vi "Read id.vi"(8 "error in (no error)":errorcluster, 11 "Electrometer in":refnum<class "Electrometer.lvclass">) -> (0 "error out":errorcluster, 2 "ElectrometerId":enum16{"", "ID1", "ID2"}(ring), 3 "Electrometer out":refnum<class "Electrometer.lvclass">)   [LabVIEW 2016]
uses:
  Electrometer.lvclass
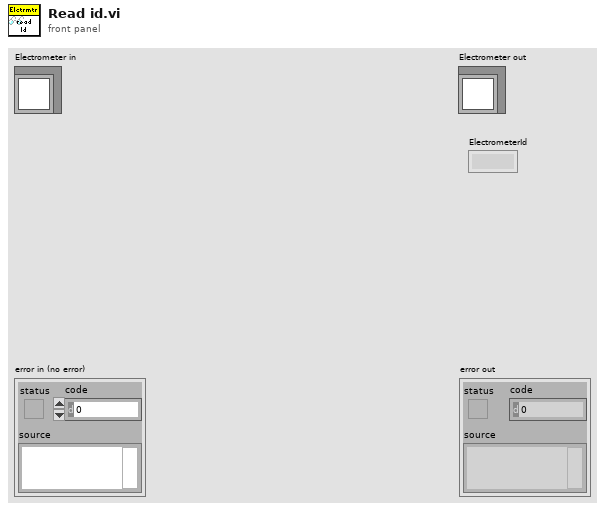
[diagram p1: front panel]
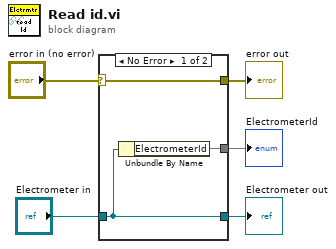
[diagram p0: block diagram]
diagram:
  n1 = case shown="No Error" "error in (no error)" {
    selector: "error in (no error)" -> [w8 w9]
    tunnel: [w8 w9] -> w4
    tunnel: [w7 w10] -> w2
    tunnel: "Electrometer in" -> [w7 w10]
    tunnel: [w6 _] -> w1
    frame No Error {
      n2 = Unbundle By Name(w7) -> ("ElectrometerId"=w6)
    }
    frame Error {
    }
  }
  "error out" <- w4
  "Electrometer out" <- w2
  "ElectrometerId" <- w1
